vi "CentroidBinning.vi"(7 "Settings.number of cam":dbl, 11 "spec cluster 3":cluster{"dp [MeV/C]":dbl[], dbl[]}[](graph)) -> (0 "spectrum":waveform(dbl), 1 "spec cluster":cluster{"xi used":dbl[], "yi":dbl[]}(graph), 2 "Charge [pC]":dbl format="%0.4f", 3 "specInfo":T1 {"Charge [pC]" format="%0.4f"}, 5 "time:specPost":u32)   [LabVIEW 2011]
uses:
  specInfo_TypDef.ctl
  NI_Gmath.lvlib
  NI_AAL_SigProc.lvlib
  NI_AALPro.lvlib
  NI_AALBase.lvlib
panel:
  out "spec cluster 2":cluster{dbl[], dbl[]}[](graph)
  out "peak energy (min)":dbl
  out "peak energy (max)":dbl
  out "mean":dbl
  out "fractional index or x":dbl
  out "max energy (10% of max counts)":dbl
  out "yi":dbl[](array[numeric]) format="%_6g"
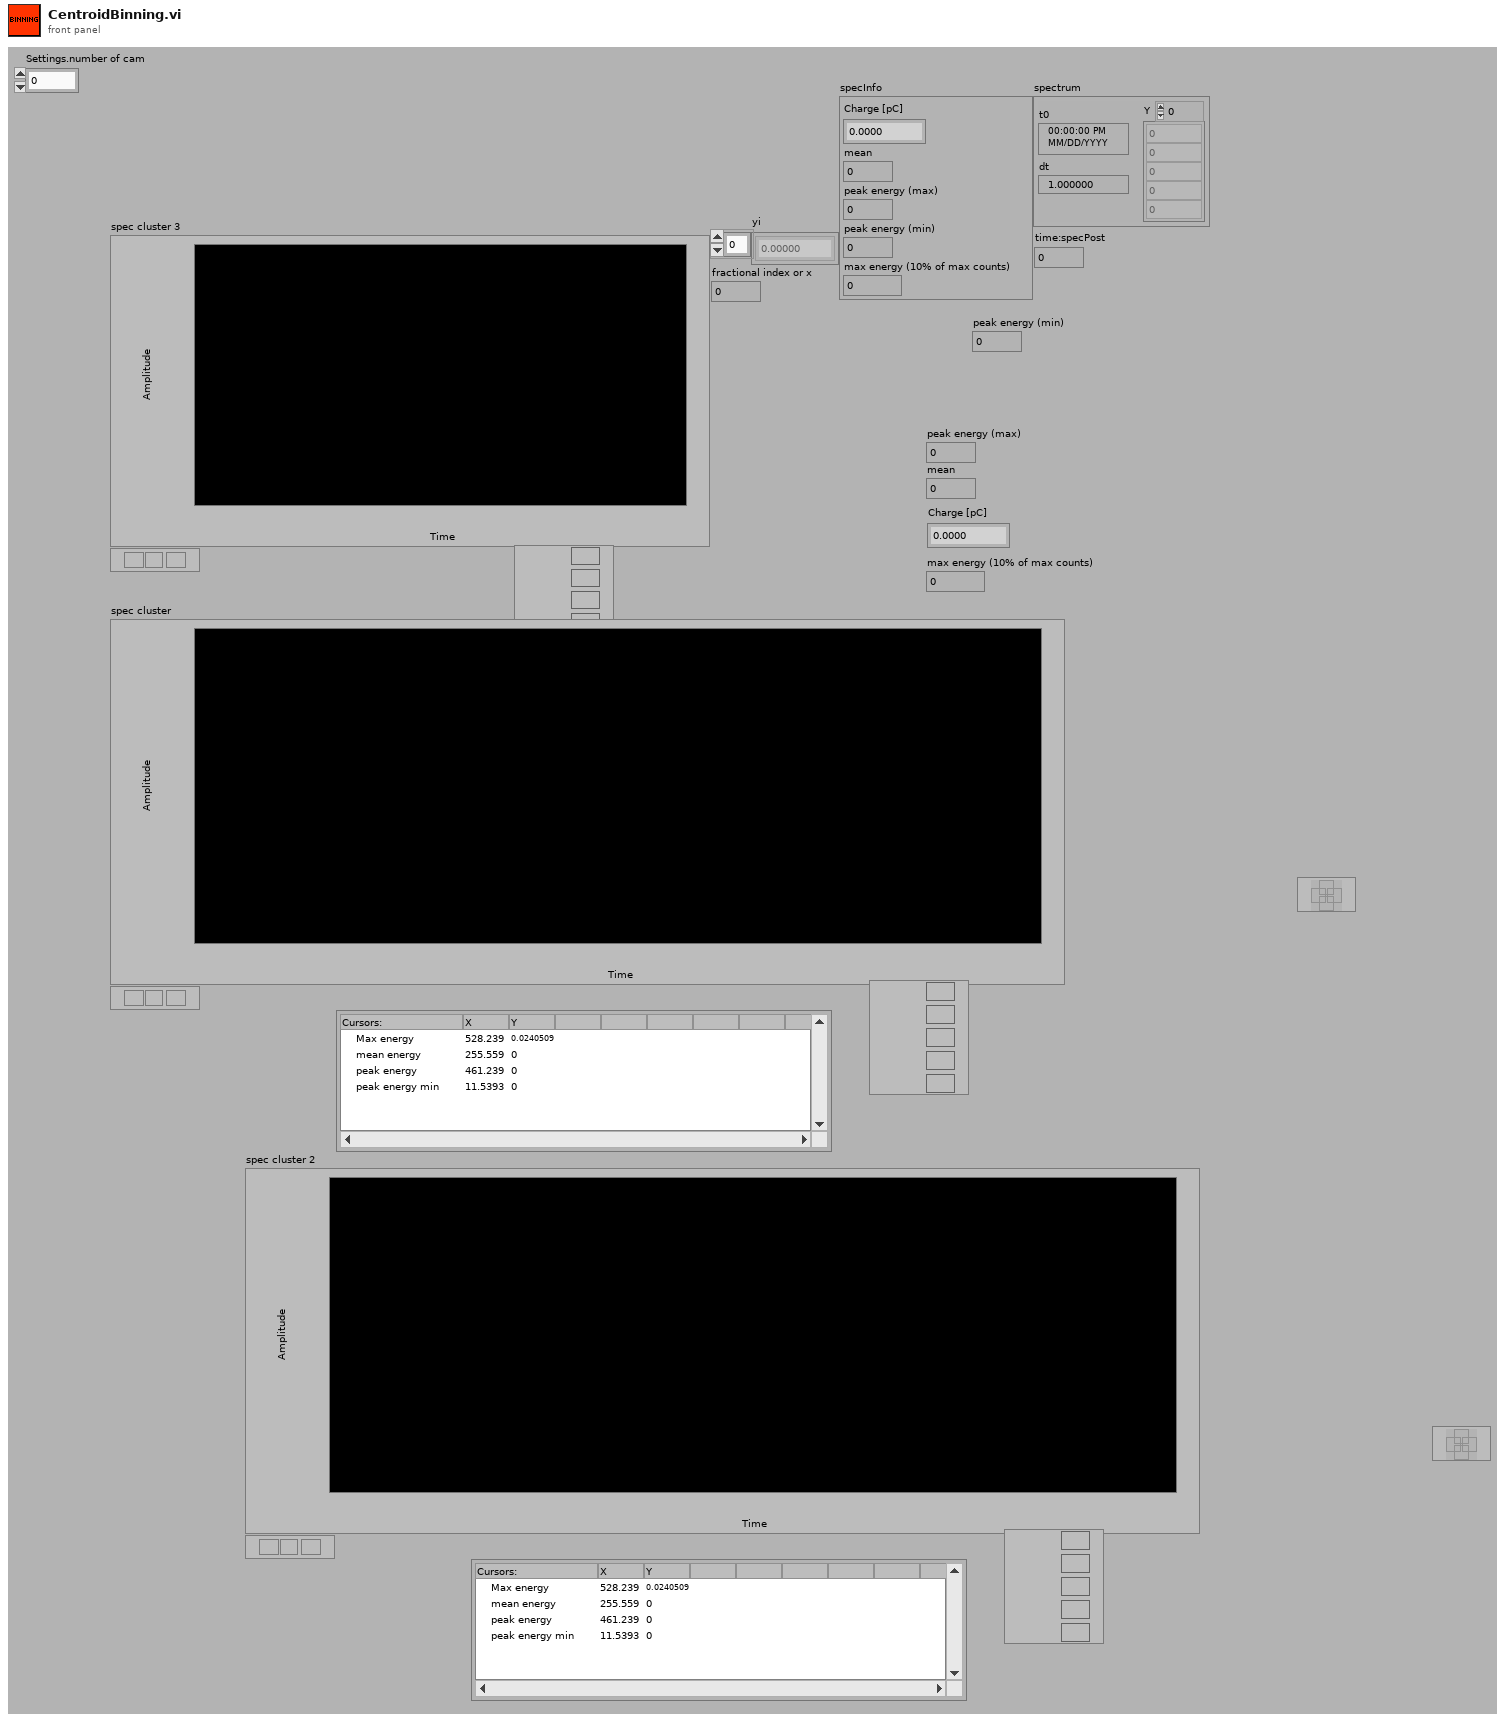
[diagram p1: front panel]
types:
  T1 = typedef "specInfo_TypDef.ctl" = cluster{"Charge [pC]":dbl, "mean":dbl, "peak energy (max)":dbl, "peak energy (min)":dbl, "max energy (10% of max counts)":dbl}
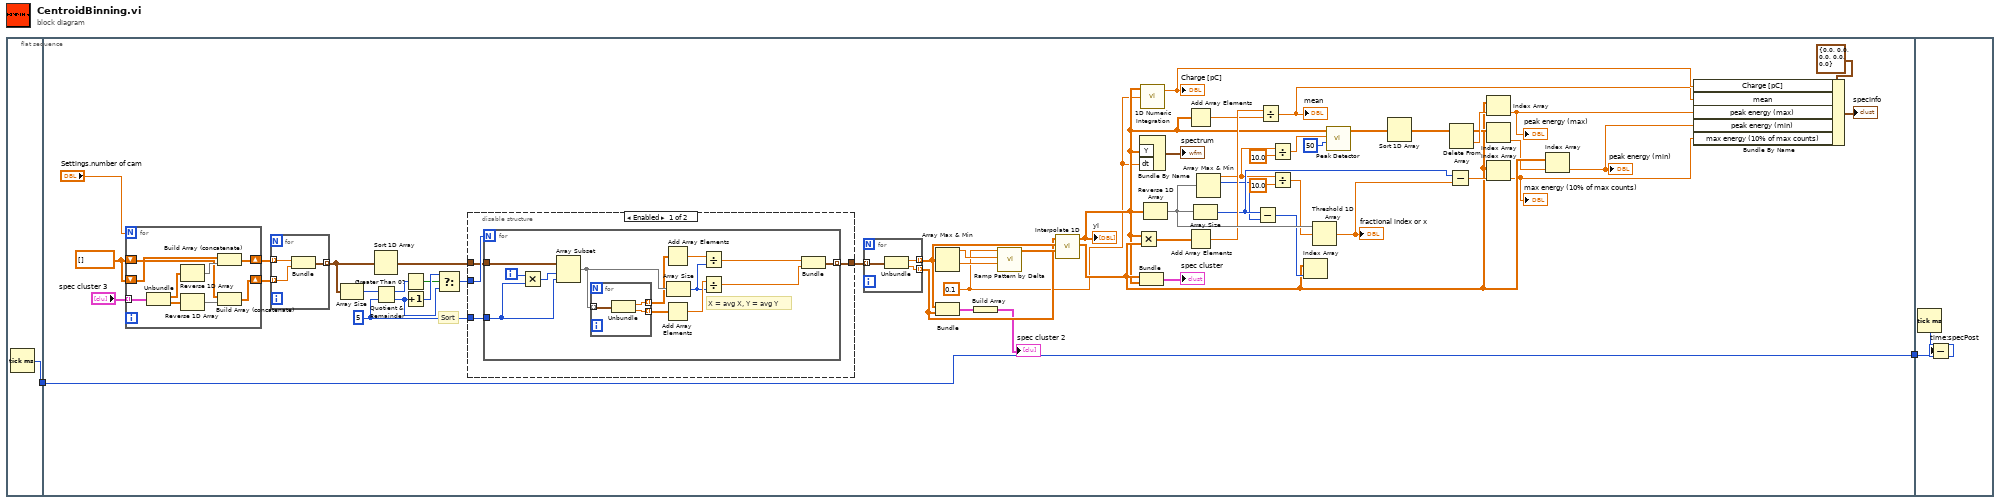
[diagram p0: block diagram]
diagram:
  n1 = flat-sequence {
    tunnel: [w3] -> w1
    tunnel: [w6] -> w2
    tunnel: w1 -> [w6]
    tunnel: w2 -> [w96]
    frame #0 {
      n2 = Tick Count (ms)() -> (millisecond timer value=w3:u32)
    }
    frame #1 {
      w8 = 0.1 ("delta")
      w47 = dbl[] []
      w54 = 5 ("Samples/bin")
      # "Sort"
      n3 = for {
        N: "Settings.number of cam" -> [_]
        tunnel: "spec cluster 3" -> [w88] mode=indexing
        shift-right: [w85] -> w46
        shift-left: w47 -> [w84]
        shift-right: [w81] -> w40
        shift-left: w47 -> [w80]
        n4 = Unbundle(w88) -> ("dp [MeV/C]"=w87:dbl[], w83:dbl[])
        n5 = Reverse 1D Array(array=w87) -> (reversed array=w86:dbl[])
        n6 = Reverse 1D Array(array=w83) -> (reversed array=w82:dbl[])
        n7 = Build Array (concatenate)(w84, w86) -> (w85:dbl[])
        n8 = Build Array (concatenate)(w80, w82) -> (w81:dbl[])
      }
      n9 = for {
        tunnel: w46 -> [w94] mode=indexing
        tunnel: w40 -> [w93] mode=indexing
        tunnel: [w92] -> w51 mode=indexing
        n10 = Bundle(w94, w93) -> (w92:cluster{dbl, dbl})  [unwired: 1 in]
      }
      n11 = Array Size(array=w51) -> (size(s)=w52:i32)
      n12 = Sort 1D Array(array=w51) -> (sorted array=w49:cluster{dbl, dbl}[])
      n13 = Quotient & Remainder(x=w52, y=w54) -> (x-y*floor(x/y)=w58:i32, floor(x/y)=w56:i32)
      n14 = Greater Than 0?(x=w58) -> (x > 0?=w55:bool)
      n15 = Increment(x=w56) -> (x+1=w57:i32)
      n16 = Select(t=w57, s=w55, f=w56) -> (s? t:f=w53:i32)
      n17 = disable-structure shown="Enabled" {
        disable-tunnel: w54 -> [w62 _]
        disable-tunnel: w53 -> [w61 _]
        disable-tunnel: [w60 w79] -> w50
        disable-tunnel: w49 -> [w59 w79]
        frame Enabled {
          n18 = for {
            N: w61 -> [_]
            tunnel: w59 -> [w75]
            tunnel: w62 -> [w73]
            tunnel: [w70] -> w60 mode=indexing
            i -> [w74]
            # "X = avg X, Y = avg Y"
            n19 = Multiply(x=w74, y=w73) -> (x*y=w72:i32)
            n20 = Array Subset(array=w75, index=w72, length=w73) -> (w71:cluster{dbl, dbl}[])
            n21 = for {
              tunnel: w71 -> [w78] mode=indexing
              tunnel: [w77] -> w69 mode=indexing
              tunnel: [w76] -> w68 mode=indexing
              n22 = Unbundle(w78) -> (w77:dbl, w76:dbl)
            }
            n23 = Add Array Elements(numeric array=w69) -> (sum=w66:dbl)
            n24 = Add Array Elements(numeric array=w68) -> (sum=w67:dbl)
            n25 = Array Size(array=w71) -> (size(s)=w65:i32)
            n26 = Divide(x=w66, y=w65) -> (x/y=w64:dbl)
            n27 = Divide(x=w67, y=w65) -> (x/y=w63:dbl)
            n28 = Bundle(w64, w63) -> (w70:cluster{dbl, dbl})  [unwired: 1 in]
          }
        }
        frame Disabled {
        }
      }
      n29 = for {
        tunnel: w50 -> [w91] mode=indexing
        tunnel: [w90] -> w42 mode=indexing
        tunnel: [w89] -> w41 mode=indexing
        n30 = Unbundle(w91) -> (w90:dbl, w89:dbl)
      }
      n31 = Array Max & Min(array=w42) -> (max value=w44:dbl, min value=w45:dbl)  [unwired: 2 out]
      n32 = Bundle(w42, w41) -> (w39:cluster{dbl[], dbl[]})  [unwired: 1 in]
      n33 = Build Array(w39) -> (→"spec cluster 2":cluster{dbl[], dbl[]}[])
      n34 = call "Ramp Pattern by Delta.vi"("start"=w45, "end"=w44, "delta"=w8) -> ("Ramp Pattern"=w43:dbl[])  [unwired: 6 in, 2 out]
      n35 = call "Interpolate 1D.vi"("xi"=w43, "X"=w42, "Y"=w41) -> ("xi used"=w18:dbl[], "yi"=w9:dbl[])  [unwired: 6 in, 1 out]
      "yi" <- w9
      n36 = Multiply(x=w9, y=w18) -> (x*y=w32:dbl[])
      n37 = Bundle By Name("Y"=w9, "dt"=w8) -> (→"spectrum":waveform(dbl))  [unwired: 1 in]
      n38 = Bundle("xi used"=w18, "yi"=w9) -> (→"spec cluster":cluster{"xi used":dbl[], "yi":dbl[]})  [unwired: 1 in]
      n39 = call "1D Numeric Integration.vi"("dt"=w8, "Input Array"=w9) -> ("result"=w15:dbl)  [unwired: 1 in, 1 out]
      "Charge [pC]" <- w15
      n40 = Reverse 1D Array(array=w9) -> (reversed array=w37:dbl[])
      n41 = Add Array Elements(numeric array=w9) -> (sum=w30:dbl)
      n42 = Add Array Elements(numeric array=w32) -> (sum=w31:dbl)
      n43 = Array Size(array=w37) -> (size(s)=w29:i32)
      n44 = Array Max & Min(array=w37) -> (max value=w26:dbl, max index (indices)=w28:i32)  [unwired: 2 out]
      n45 = Subtract(x=w29, y=w28) -> (x-y=w27:i32)
      n46 = Divide(x=w31, y=w30) -> (x/y=w14:dbl)
      "mean" <- w14
      n47 = Divide(x=w26, y=10.0) -> (x/y=w24:dbl)
      n48 = Divide(x=w26, y=10.0) -> (x/y=w33:dbl)
      n49 = Index Array(array=w18, index=w27) -> ()  [unwired: 1 out]
      n50 = Threshold 1D Array(2:w33, 3:w37) -> (0:w36:dbl)  [unwired: 1 in]
      "fractional index or x" <- w36
      n51 = call "Peak Detector.vi"("width"=50, "threshold"=w24, "X"=w9) -> ("Locations"=w22:dbl[])  [unwired: 4 in, 4 out]
      n52 = Sort 1D Array(array=w22) -> (sorted array=w21:dbl[])
      n53 = Subtract(x=w29, y=w36) -> (x-y=w34:dbl)
      n54 = Delete From Array(array=w21) -> (deleted portion=w20:dbl, array with subset deleted=w19:dbl[])  [unwired: 2 in]
      n55 = Index Array(array=w18, index=w20) -> (element=w13:dbl)
      "peak energy (max)" <- w13
      n56 = Index Array(array=w19) -> (element=w17:dbl)  [unwired: 1 in]
      n57 = Index Array(array=w18, index=w34) -> (element=w11:dbl)
      "max energy (10% of max counts)" <- w11
      n58 = Index Array(array=w18, index=w17) -> (element=w12:dbl)
      "peak energy (min)" <- w12
      n59 = Bundle By Name(cluster=T1 {"Charge [pC]"=0.0, "mean"=0.0, "peak energy (max)"=0.0, "peak energy (min)"=0.0, "max energy (10% of max counts)"=0.0} ("specInfo"), "Charge [pC]"=w15, "mean"=w14, "peak energy (max)"=w13, "peak energy (min)"=w12, "max energy (10% of max counts)"=w11) -> (→"specInfo":T1)
    }
    frame #2 {
      n60 = Tick Count (ms)() -> (millisecond timer value=w97:u32)
      n61 = Subtract(x=w97, y=w96) -> (x-y=→"time:specPost":u32)
    }
  }
